vi "VI Tree.vi"() -> ()   [LabVIEW 2013, in "QWTBLVLib.lvlib"]
doc: "This is the instrument driver for the Agilent 34401/34410/34411 digital multimeter."
uses:
  QWTBLVLib.lvlib
  TD Quantity.ctl
  TD Algorithm Information.ctl
  TD Uncertainty Calculation Method.ctl
  TD Correlation Calculation Settings.ctl
  TD DOF Calculation Settings.ctl
  TD MCM Calculation Method.ctl
  TD MCM Calculation Settings.ctl
  TD Calculation Settings.ctl
  TD Algorithm Information Output.ctl
  TD Algorithm Information Input.ctl
panel:
  out "Data Out":T1[](array[typedef])
  out "Quantity":T1={"Name"="A", "Value"=[[1.0]], "Uncertainty"=[[1.0]], "Degrees of\nFreedom"=[[10.0]], "Correlation"=[[10.0]], "Randomized uncertainty"=[[10.0]]}
  # "SEE DIAGRAM\nFOR VI Tree"
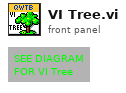
[diagram p1: front panel]
types:
  T1 = typedef "QWTBLVLib.lvlib/TD Quantity.ctl" = cluster{"Name":string, "Value":dbl[][], "Uncertainty":dbl[][], "Degrees of\nFreedom":dbl[][], "Correlation":dbl[][], "Randomized uncertainty":dbl[][]}
  T2 = typedef "QWTBLVLib.lvlib/TD Calculation Settings.ctl" = cluster{"Strict":bool, "Verbose":bool, "Uncertainty Calculation Method":T3, "Correlations":T4, "Degrees of Freedom":T5, "MCM Calculation Settings":T6}
  T3 = typedef "QWTBLVLib.lvlib/TD Uncertainty Calculation Method.ctl" = enum16{"none", "GUF", "MCM"}
  T4 = typedef "QWTBLVLib.lvlib/TD Correlation Calculation Settings.ctl" = cluster{"Required":bool, "Generate":bool}
  T5 = typedef "QWTBLVLib.lvlib/TD DOF Calculation Settings.ctl" = cluster{"Required":bool, "Generate":bool}
  T6 = typedef "QWTBLVLib.lvlib/TD MCM Calculation Settings.ctl" = cluster{"Repeats":i32, "Verbose":bool, "Parallelization method":T7, "Processors":i32, "Temporary directory":string, "Randomize":bool}
  T7 = typedef "QWTBLVLib.lvlib/TD MCM Calculation Method.ctl" = enum16{"Single Core", "Multi Core", "Multi Station"}
  T8 = typedef "QWTBLVLib.lvlib/TD Algorithm Information.ctl" = cluster{"ID":string, "Name":string, "Description":string, "Citation":string, "Remarks":string, "License":string, "Inputs":T9[], "Outputs":T10[], "Provides GUF":bool, "Provides MCM":bool, "Full path":string}
  T9 = typedef "QWTBLVLib.lvlib/TD Algorithm Information Input.ctl" = cluster{"Name":string, "Description":string, "Alternative":i32, "Optional":i32, "Parameter":i32}
  T10 = typedef "QWTBLVLib.lvlib/TD Algorithm Information Output.ctl" = cluster{"Name":string, "Description":string}
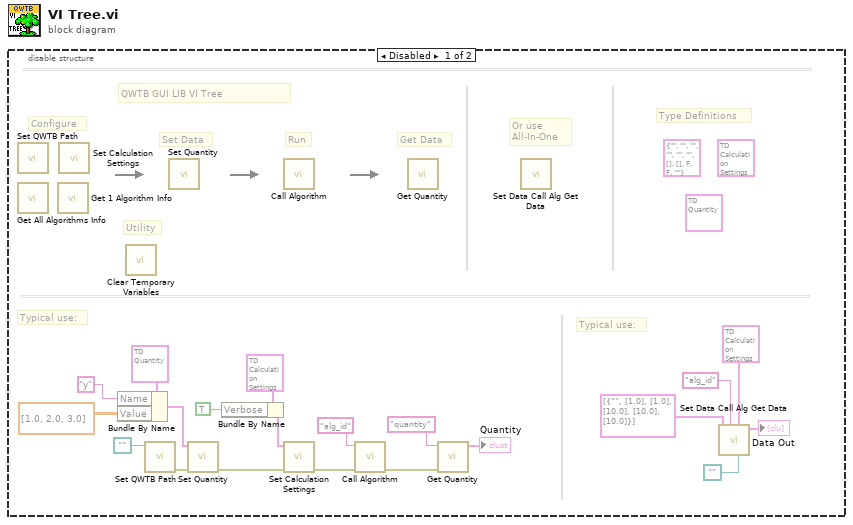
[diagram p0: block diagram]
diagram:
  n1 = disable-structure shown="Disabled" {
    frame Disabled {
      (unwired) T1 {"Name"="", "Value"=[[1.0]], "Uncertainty"=[[1.0]], "Degrees of\nFreedom"=[[10.0]], "Correlation"=[[10.0]], "Randomized uncertainty"=[[10.0]]} ("Quantity")
      (unwired) T2 {"Strict"=FALSE, "Verbose"=FALSE, "Uncertainty Calculation Method"=enum."none", "Correlations"={"Required"=FALSE, "Generate"=FALSE}, "Degrees of Freedom"={"Required"=FALSE, "Generate"=FALSE}, "MCM Calculation Settings"={"Repeats"=0, "Verbose"=FALSE, "Parallelization method"=enum."Single Core", "Processors"=0, "Temporary directory"="", "Randomize"=FALSE}} ("Calculation Settings")
      (unwired) T8 {"ID"="", "Name"="", "Description"="", "Citation"="", "Remarks"="", "License"="", "Inputs"=[], "Outputs"=[], "Provides GUF"=FALSE, "Provides MCM"=FALSE, "Full path"=""} ("Algorithm Information")
      # "Typical use:"
      # "Typical use:"
      # "QWTB GUI LIB VI Tree"
      # "Type Definitions"
      # "Set Data"
      # "Or use\nAll-In-One"
      # "Configure"
      # "Utility"
      # "Get Data"
      # "Run"
      n2 = call "Set QWTB Path.vi"() -> ()  [unwired: 11 in, 1 out]
      n3 = call "Get All Algorithms Info.vi"() -> ()  [unwired: 10 in, 2 out]
      n4 = call "Get 1 Algorithm Info.vi"() -> ()  [unwired: 10 in, 2 out]
      n5 = call "Set Calculation Settings.vi"() -> ()  [unwired: 11 in, 1 out]
      n6 = Bundle By Name(cluster=T1 {"Name"="", "Value"=[[1.0]], "Uncertainty"=[[1.0]], "Degrees of\nFreedom"=[[10.0]], "Correlation"=[[10.0]], "Randomized uncertainty"=[[10.0]]} ("Quantity"), "Name"="y", "Value"=dbl[][] [[1.0, 2.0, 3.0]]) -> (w12:T1)
      n7 = call "Clear Temporary Variables.vi"() -> ()  [unwired: 11 in, 1 out]
      n8 = call "Set QWTB Path.vi"("QWTB Folder Path"=path "") -> ("error out"=w20:errorcluster)  [unwired: 10 in]
      n9 = call "Set Quantity.vi"() -> ()  [unwired: 11 in, 1 out]
      n10 = call "Set Quantity.vi"("error in"=w20, "Quantity"=w12) -> ("error out"=w19:errorcluster)  [unwired: 9 in]
      n11 = Bundle By Name(cluster=T2 {"Strict"=FALSE, "Verbose"=FALSE, "Uncertainty Calculation Method"=enum."none", "Correlations"={"Required"=FALSE, "Generate"=FALSE}, "Degrees of Freedom"={"Required"=FALSE, "Generate"=FALSE}, "MCM Calculation Settings"={"Repeats"=0, "Verbose"=FALSE, "Parallelization method"=enum."Single Core", "Processors"=0, "Temporary directory"="", "Randomize"=FALSE}} ("Calculation Settings"), "Verbose"=TRUE) -> (w10:T2)
      n12 = call "Call Algorithm.vi"() -> ()  [unwired: 11 in, 1 out]
      n13 = call "Set Calculation Settings.vi"("error in"=w19, "Calculation Settings"=w10) -> ("error out"=w18:errorcluster)  [unwired: 9 in]
      n14 = call "Call Algorithm.vi"("error in"=w18, "Algorithm ID"="alg_id") -> ("error out"=w17:errorcluster)  [unwired: 9 in]
      n15 = call "Get Quantity.vi"() -> ()  [unwired: 10 in, 2 out]
      n16 = call "Get Quantity.vi"("error in"=w17, "Quantity Name"="quantity") -> ("Quantity"=→"Quantity":T1)  [unwired: 8 in, 1 out]
      n17 = call "Set Data Call Alg Get Data.vi"() -> ()  [unwired: 10 in, 2 out]
      n18 = call "Set Data Call Alg Get Data.vi"("QWTB Folder Path"=path "", "Calculation Settings"=T2 {"Strict"=FALSE, "Verbose"=FALSE, "Uncertainty Calculation Method"=enum."none", "Correlations"={"Required"=FALSE, "Generate"=FALSE}, "Degrees of Freedom"={"Required"=FALSE, "Generate"=FALSE}, "MCM Calculation Settings"={"Repeats"=0, "Verbose"=FALSE, "Parallelization method"=enum."Single Core", "Processors"=0, "Temporary directory"="", "Randomize"=FALSE}}, "Algorithm ID"="alg_id", "Data In"=T1[] [{"Name"="", "Value"=[[1.0]], "Uncertainty"=[[1.0]], "Degrees of\nFreedom"=[[10.0]], "Correlation"=[[10.0]], "Randomized uncertainty"=[[10.0]]}]) -> ("Data Out"=→"Data Out":T1[])  [unwired: 6 in, 1 out]
    }
    frame Enabled {
    }
  }
